vi "Stop.vi"(8 "error in (no error)":errorcluster, 11 "CameraStream in":refnum<class "CameraStream.lvclass">) -> (0 "error out":errorcluster, 3 "CameraStream (Duplicate)":refnum<class "CameraStream.lvclass">)   [LabVIEW 2020, in "g_ar_toolkit.capture.lvlib" / "CameraStream.lvclass"]
uses:
  CameraStream.lvclass
  CameraStream.lvclass/CameraStream.ctl
  g_ar_toolkit.common/g_ar_toolkit.common.lvlib
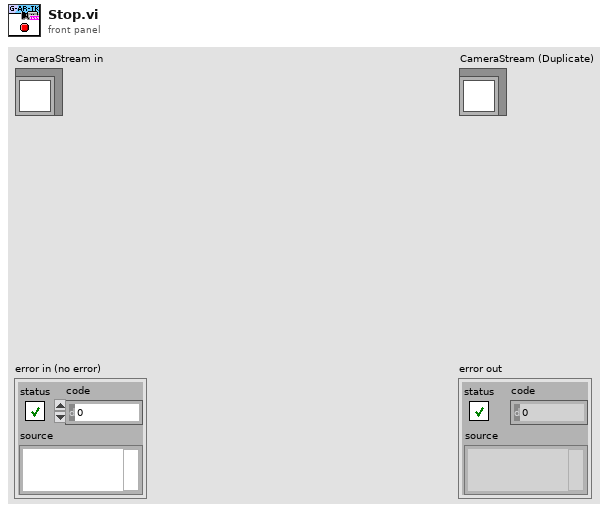
[diagram p1: front panel]
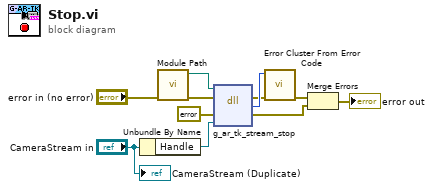
[diagram p0: block diagram]
diagram:
  n1 = Unbundle By Name("CameraStream in") -> ("Handle"=w10:refnum<data-value>)
  n2 = call "Module Path.vi"("error in (no error)"="error in (no error)") -> ("error out"=w2:errorcluster, "Path"=w1:path)  [unwired: 9 in]
  n3 = dll-call lib="?" fn="g_ar_tk_stream_stop"(path in=w1, error in=w2, "error_cluster"=errorcluster {"status"=FALSE, "code"=0, "source"=""} ("error constant"), "EDVR_strm"=w10) -> (error out=w7:errorcluster, "MgErr"=w8:i32, "error_cluster"=w4:errorcluster)  [unwired: 2 in, 1 out]
  n4 = call <vilib>:"Error Cluster From Error Code.vi"("error in (no error)"=w7, "error code (0)"=w8) -> ("error out"=w6:errorcluster)  [unwired: 7 in]
  n5 = Merge Errors(w6, w4) -> (→"error out":errorcluster)
  "CameraStream (Duplicate)" <- "CameraStream in"
